vi "MRC Alert Get Alert Text.vi"(8 "error in (no error)":errorcluster, 11 "handle":i64) -> (0 "error out":errorcluster, 2 "text":T1)   [LabVIEW 2026, in "MrcLib.lvlib"]
doc: "MRC_Status MRC_CALLCONV MRC_Alert_GetAlertText(MRC_AlertHandle handle,\n struct MRC_String* text);"
uses:
  MrcLib.lvlib
  MrcLib.dll
  <vilib>/MRC/Types/MRC String.ctl
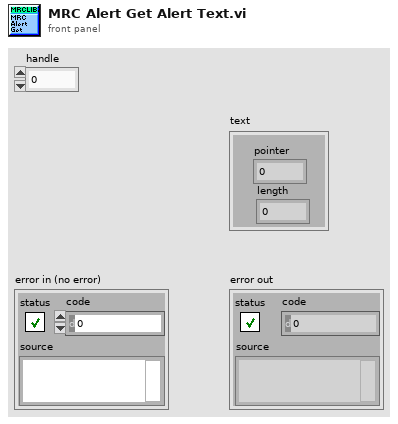
[diagram p1: front panel]
types:
  T1 = typedef "MRC String.ctl" = cluster{"pointer":u64, "length":u64}
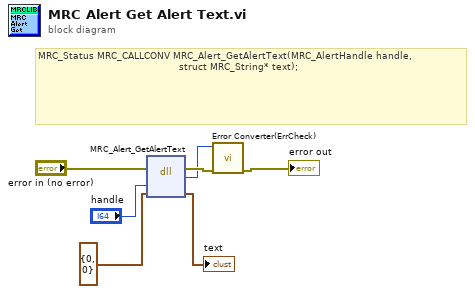
[diagram p0: block diagram]
diagram:
  # "MRC_Status MRC_CALLCONV MRC_Alert_GetAlertText(MRC_AlertHandle handle,\n                                               struct MRC_String* text);"
  n1 = dll-call lib="MrcLib.*" fn="MRC_Alert_GetAlertText"(error in="error in (no error)", "handle"="handle", "text"=T1 {"pointer"=0, "length"=0} ("group")) -> (error out=w3:errorcluster, w1:i32, "text"=→"text":T1)  [unwired: 3 in, 1 out]
  n2 = call <vilib>:"Error Converter(ErrCheck).vi"("error in (no error)"=w3, "status"=w1) -> ("error out"=→"error out":errorcluster)  [unwired: 9 in]
